vi "Create First VI Determine the area of the an triangle.vi"() -> ()   [LabVIEW 2024]
panel:
  out "Area (cm^2)":dbl
  in  "Height (cm)":dbl
  in  "Base (cm)":dbl
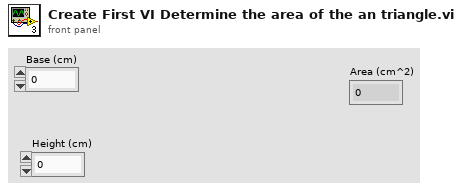
[diagram p1: front panel]
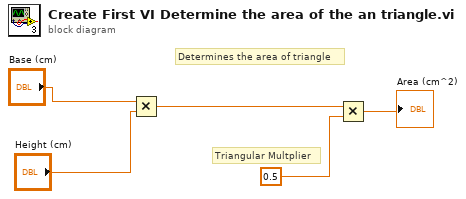
[diagram p0: block diagram]
diagram:
  # "Triangular Multplier"
  # "Determines the area of triangle"
  n1 = Multiply(x="Base (cm)", y="Height (cm)") -> (x*y=w3:dbl)
  n2 = Multiply(x=w3, y=0.5) -> (x*y=→"Area (cm^2)":dbl)
